vi "OldFashionFXPRead.vi"(8 "Error In":errorcluster) -> (0 "error out":errorcluster, 1 "Values":dbl[](array[numeric]), 3 "Average":dbl)   [LabVIEW 2018]
uses:
  <vilib>/addons/FPGA Advanced Session Resources/LVFPGA Adv Session Resources/OpenByNameSubVI.vi
  <vilib>/rvi/interface/common/dynamic/niFpgaEscapeDelimiterAndNull.vi
  <vilib>/Utility/error.llb/Error Cluster From Error Code.vi
  <vilib>/rvi/errors/niLvFpgaAdjustHostInterfaceError.vi
  <vilib>/addons/FPGA Advanced Session Resources/LVFPGA Adv Session Resources/OpenByName.xnode
  <vilib>/rvi/interface/nirviReadWriteControl/nirviReadWriteControl.xnode
  <vilib>/addons/FPGA Advanced Session Resources/LVFPGA Adv Session Resources/LVFPGAAdvSessionResources.lvlib
  NiFpgaLv.dll
  <vilib>/rvi/interface/Simulation/niFpgaSimulationCallBeginRW.vi
panel:
  out "Value":fxp<+/-,16,2>
  out "Waveform Graph":dbl[](graph)
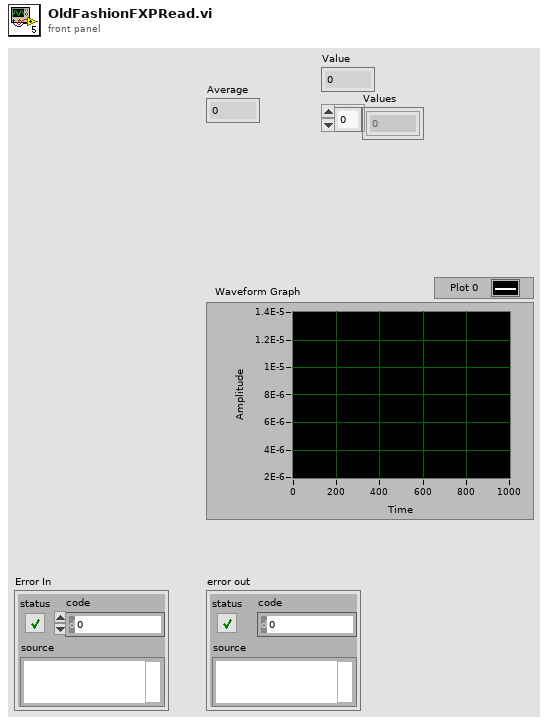
[diagram p1: front panel]
types:
  T1 = typedef "LVFPGAAdvSessionResources.lvlib/ResourceInfo.ctl" = cluster{"Resource name":string, "Data type":variant, "Resource type":enum16{"Register", "Host To Target FIFO", "Target To Host FIFO"}}
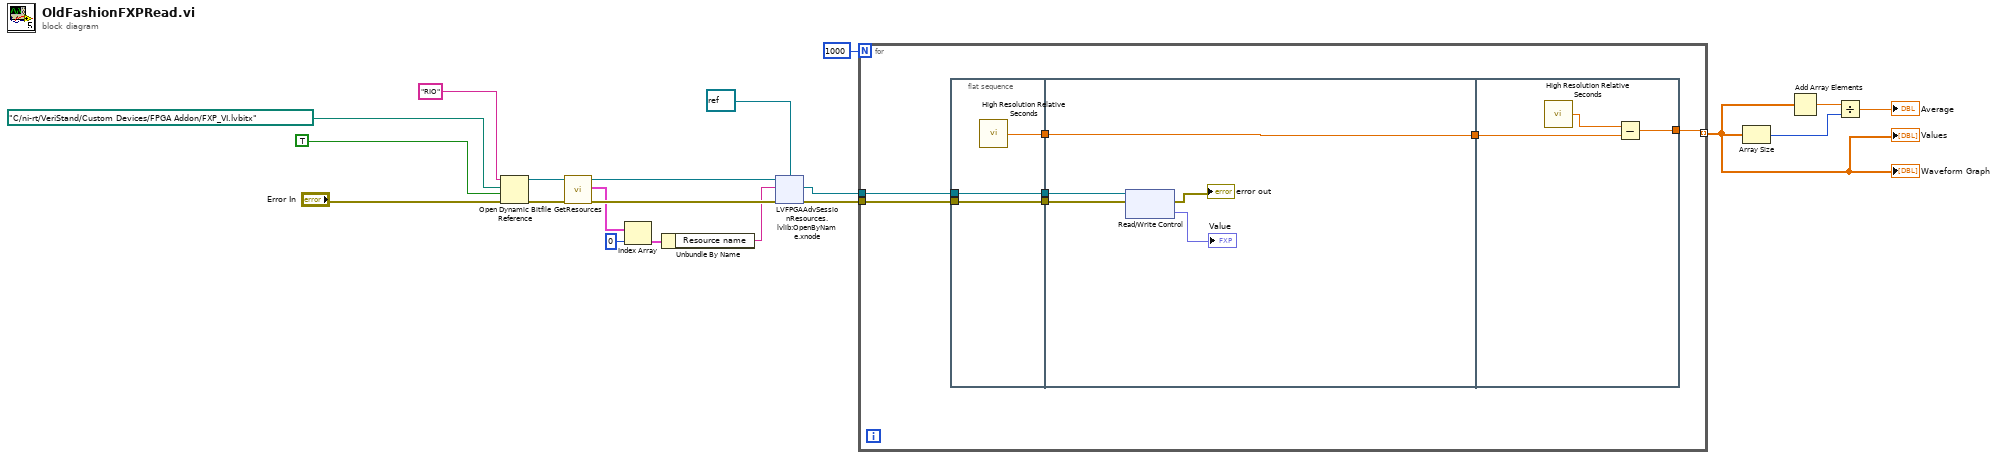
[diagram p0: block diagram]
diagram:
  n1 = Open Dynamic Bitfile Reference(0:"RIO" ("Device address"), 1:path "C:/ni-rt/VeriStand/Custom Devices/FPGA Addon/FXP_VI.lvbitx" ("Bitfile path"), 2:TRUE ("Run When Loaded"), 3:"Error In") -> (5:w7:refnum<k20>, 8:w8:errorcluster)  [unwired: 1 in]
  n2 = call <vilib>:"GetResources.vi"("error in (no error)"=w8, "FPGA VI Reference in"=w7) -> ("error out"=w6:errorcluster, "Resource info out"=w4:T1[], "FPGA VI Reference out"=w5:refnum<k20>)  [unwired: 7 in]
  n3 = Index Array(array=w4, index=0) -> (element=w2:T1)
  n4 = Unbundle By Name(w2) -> ("Resource name"=w1:string)
  n5 = xnode "LVFPGAAdvSessionResources.lvlib:OpenByName.xnode"("FPGA VI Reference in"=w5, "Resource name in"=w1, "Single resource reference type in"=refnum<k20> refnum, "Error in"=w6) -> ("Single resource reference out"=w9:refnum<k20>, "Error out"=w10:errorcluster)  [unwired: 1 out]
  n6 = for {
    N: 1000 -> [_]
    tunnel: [w25] -> w17 mode=indexing
    tunnel: w10 -> [w24]
    tunnel: w9 -> [w22]
    n7 = flat-sequence {
      tunnel: [w30] -> w27
      tunnel: w24 -> [w29]
      tunnel: [w29] -> w23
      tunnel: w22 -> [w28]
      tunnel: [w28] -> w21
      tunnel: w27 -> [w35]
      tunnel: [w35] -> w26
      tunnel: w23 -> [w34]
      tunnel: w21 -> [w33]
      tunnel: w26 -> [w37]
      tunnel: [w36] -> w25
      frame #0 {
        n8 = call <vilib>:"High Resolution Relative Seconds.vi"() -> ("relative seconds"=w30:dbl)
      }
      frame #1 {
        n9 = xnode "Read/Write Control"("FPGA VI Reference In"=w33, "error in"=w34) -> ("error out"=→"error out":errorcluster, "Value"=→"Value":fxp<+/-,16,2>)  [unwired: 1 out]
      }
      frame #2 {
        n10 = call <vilib>:"High Resolution Relative Seconds.vi"() -> ("relative seconds"=w38:dbl)
        n11 = Subtract(x=w38, y=w37) -> (x-y=w36:dbl)
      }
    }
  }
  "Waveform Graph" <- w17
  "Values" <- w17
  n12 = Array Size(array=w17) -> (size(s)=w19:i32)
  n13 = Add Array Elements(numeric array=w17) -> (sum=w20:dbl)
  n14 = Divide(x=w20, y=w19) -> (x/y=→"Average":dbl)
